vi "Pixel integration - Pixel begin and duration.vi"(8 "error in (no error)":errorcluster, 9 "duration, (ps)":i64=1000, 10 "pixel_start_ch":i32, 11 "tagger in":refnum<k24>) -> (0 "error out":errorcluster, 1 "pixel_end_ch":i32, 2 "pixel_start_ch":i32, 3 "delayed channel out":refnum<k24>)   [LabVIEW 2014]
uses:
  SwabianInstruments.TimeTagger
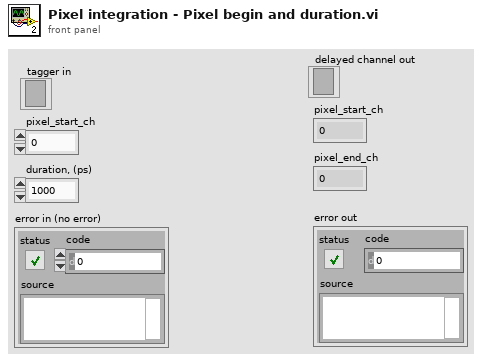
[diagram p1: front panel]
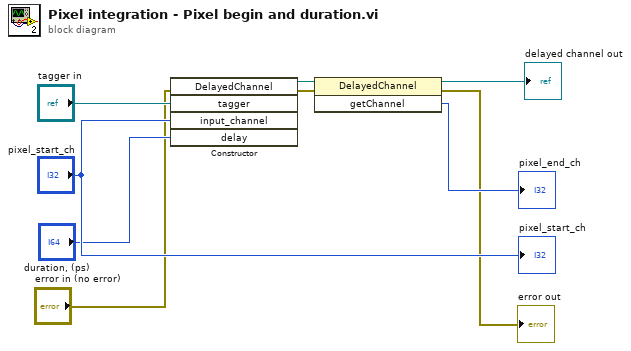
[diagram p0: block diagram]
diagram:
  n1 = constructor class="DelayedChannel"(error in="error in (no error)", "tagger"="tagger in", "input_channel"="pixel_start_ch", "delay"="duration, (ps)") -> (reference out=w6:refnum<k24>, error out=w7:errorcluster)  [unwired: 2 in, 4 out]
  n2 = invoke class="DelayedChannel" method="getChannel"(reference=w6, error in=w7) -> (reference out=→"delayed channel out":refnum<k24>, error out=→"error out":errorcluster, "getChannel"=→"pixel_end_ch":i32)  [unwired: 1 in]
  "pixel_start_ch" <- "pixel_start_ch"
